vi "FGV_TE Controller.vi"(7 "Operation (Read)":T4, 8 "error in (no error)":errorcluster, 11 "FGV_TEC_IN":T1={"SVs"={"Unused"=0.0}, "PVs"={"FW & HW Versions"={"Device Type [I32]"=0, "Device Type [String]"="", "Firmware Version [I32]"=0, "Firmware Version [String]"="", "Hardware Version [I32]"=0, "Hardware Version [String]"="", "Serial No."=0}, "TEC Configuration"={"VISA resource name"="", "Device Address"=2}, "Object Target Temperature Source_CH1"=0, "Object Target Temperature Source_CH2"=0}, "Front Panel References"={"Main Loop Queue"=refnum, "meTEC_Device Type"=refnum, "meTEC_Serial No."=refnum, "meTEC_Hardware Version"=refnum, "meTEC_Firmware Version"=refnum, "meTEC_CH1_Object Target Temperature (ID 3000 / 50012) [°C]"=refnum, "meTEC_CH1_Live Set Current (ID 50001) [A]"=refnum, "meTEC_CH1_Live Set Voltage (ID 50002) [V]"=refnum, "meTEC_CH1_Live Enable (ID 50000)"=refnum, "meTEC_CH1_Input Selection (ID 2000)"=refnum, "meTEC_CH1_Object Target Temp. Source Sel. (ID 50011)"=refnum, "meTEC_CH2_Object Target Temperature (ID 3000 / 50012) [°C]"=refnum, "meTEC_CH2_Live Set Current (ID 50001) [A]"=refnum, "meTEC_CH2_Live Set Voltage (ID 50002) [V]"=refnum, "meTEC_CH2_Live Enable (ID 50000)"=refnum, "meTEC_CH2_Input Selection (ID 2000)"=refnum, "meTEC_CH2_Object Target Temp. Source Sel. (ID 50011)"=refnum, "meTEC_CH2_Object Temperature [°C]"=refnum, "meTEC_CH2_Sink Temperature [°C]"=refnum, "meTEC_CH2_Act. Output Current [A]"=refnum, "meTEC_CH2_Act. Output Voltage [V]"=refnum, "meTEC_CH2_Temperature Stability"=refnum, "Monitor Chart_CH2"=refnum, "meTEC_Initialize Device"=refnum}} caption="FGV_Rs Analyses_In") -> (0 "error out":errorcluster, 3 "FGV_TEC_OUT":T1={"SVs"={"Unused"=0.0}, "PVs"={"FW & HW Versions"={"Device Type [I32]"=0, "Device Type [String]"="", "Firmware Version [I32]"=0, "Firmware Version [String]"="", "Hardware Version [I32]"=0, "Hardware Version [String]"="", "Serial No."=0}, "TEC Configuration"={"VISA resource name"="", "Device Address"=2}, "Object Target Temperature Source_CH1"=0, "Object Target Temperature Source_CH2"=0}, "Front Panel References"={"Main Loop Queue"=refnum, "meTEC_Device Type"=refnum, "meTEC_Serial No."=refnum, "meTEC_Hardware Version"=refnum, "meTEC_Firmware Version"=refnum, "meTEC_CH1_Object Target Temperature (ID 3000 / 50012) [°C]"=refnum, "meTEC_CH1_Live Set Current (ID 50001) [A]"=refnum, "meTEC_CH1_Live Set Voltage (ID 50002) [V]"=refnum, "meTEC_CH1_Live Enable (ID 50000)"=refnum, "meTEC_CH1_Input Selection (ID 2000)"=refnum, "meTEC_CH1_Object Target Temp. Source Sel. (ID 50011)"=refnum, "meTEC_CH2_Object Target Temperature (ID 3000 / 50012) [°C]"=refnum, "meTEC_CH2_Live Set Current (ID 50001) [A]"=refnum, "meTEC_CH2_Live Set Voltage (ID 50002) [V]"=refnum, "meTEC_CH2_Live Enable (ID 50000)"=refnum, "meTEC_CH2_Input Selection (ID 2000)"=refnum, "meTEC_CH2_Object Target Temp. Source Sel. (ID 50011)"=refnum, "meTEC_CH2_Object Temperature [°C]"=refnum, "meTEC_CH2_Sink Temperature [°C]"=refnum, "meTEC_CH2_Act. Output Current [A]"=refnum, "meTEC_CH2_Act. Output Voltage [V]"=refnum, "meTEC_CH2_Temperature Stability"=refnum, "Monitor Chart_CH2"=refnum, "meTEC_Initialize Device"=refnum}} caption="FGV_Rs Analyses_Out")   [LabVIEW 2023]
uses:
  Type Defs/FGV_Operations.ctl
  Type Defs/FGV_TE Controller.ctl
  [meerstetter engineering TE Cooling]/TypeDefs/meTEC_Configuration.ctl
  Type Defs/FGV_Front Panel References.ctl
  Type Definitions/Main Loop Queue Data.ctl
  Type Definitions/Main Loop States.ctl
panel:
  # "Input"
  # "Output"
  # "PVs = Process Values"
  # "SVs = Set values / Values to be set"
  # "PVs = Process Values"
  # "SVs = Set values / Values to be set"
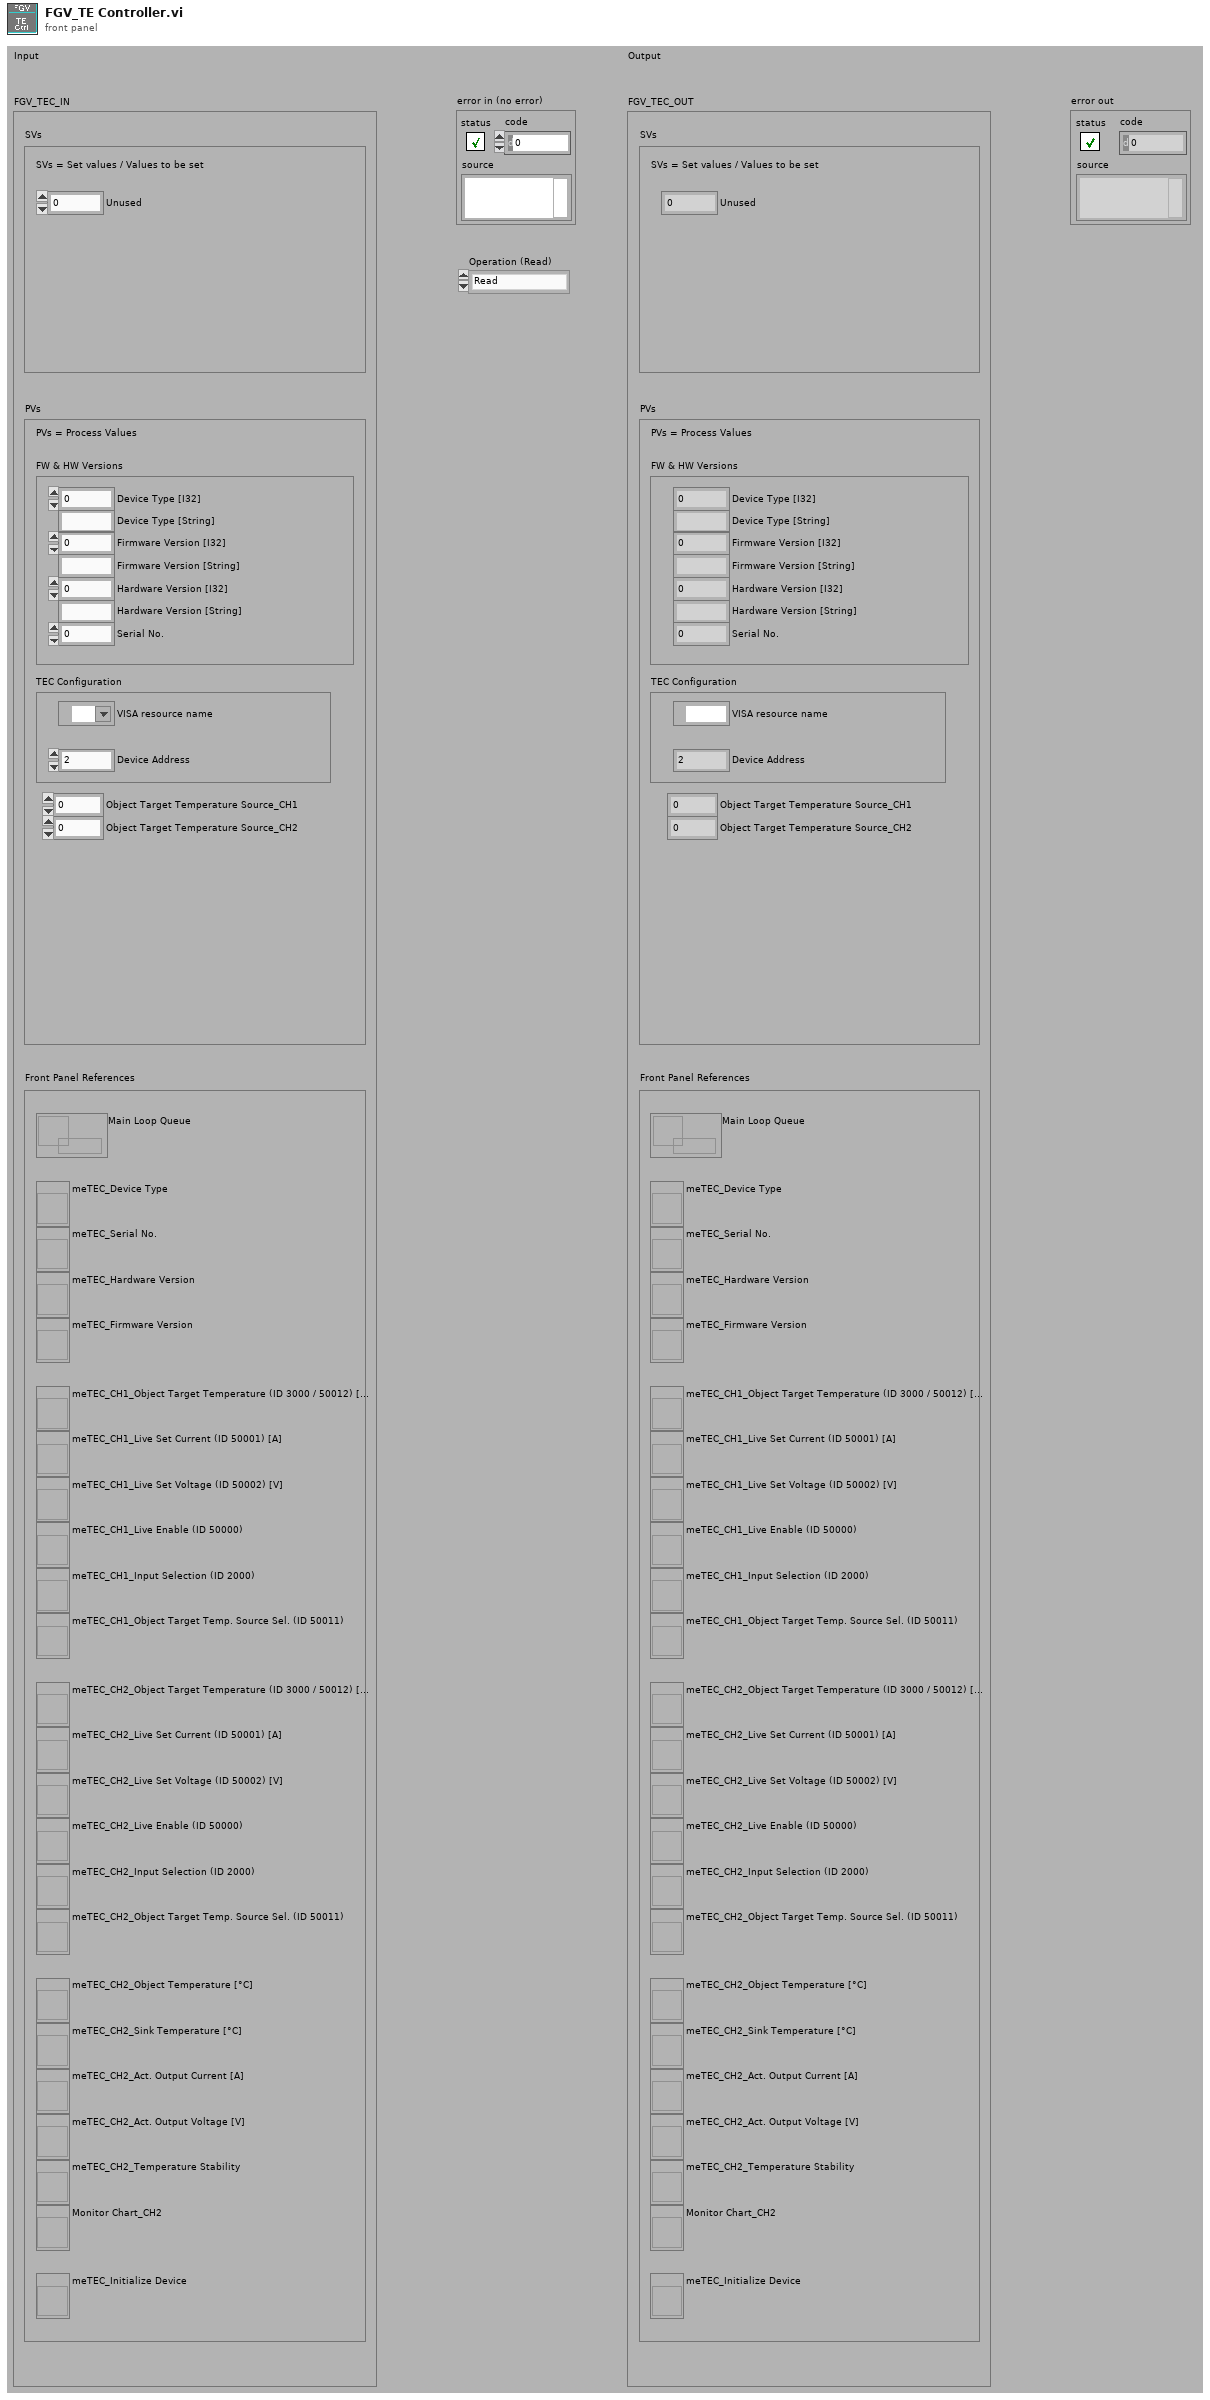
[diagram p1: front panel]
types:
  T1 = typedef "FGV_TE Controller.ctl" = cluster{"SVs":cluster{"Unused":dbl}, "PVs":cluster{"FW & HW Versions":cluster{"Device Type [I32]":i32, "Device Type [String]":string, "Firmware Version [I32]":i32, "Firmware Version [String]":string, "Hardware Version [I32]":i32, "Hardware Version [String]":string, "Serial No.":i32}, "TEC Configuration":T2, "Object Target Temperature Source_CH1":u8, "Object Target Temperature Source_CH2":u8}, "Front Panel References":T3}
  T2 = typedef "meTEC_Configuration.ctl" = cluster{"VISA resource name":refnum<visa-resource-name>, "Device Address":u16}
  T3 = typedef "FGV_Front Panel References.ctl" = cluster{"Main Loop Queue":refnum<queue>, "meTEC_Device Type":refnum<vi>, "meTEC_Serial No.":refnum<vi>, "meTEC_Hardware Version":refnum<vi>, "meTEC_Firmware Version":refnum<vi>, "meTEC_CH1_Object Target Temperature (ID 3000 / 50012) [°C]":refnum<vi>, "meTEC_CH1_Live Set Current (ID 50001) [A]":refnum<vi>, "meTEC_CH1_Live Set Voltage (ID 50002) [V]":refnum<vi>, "meTEC_CH1_Live Enable (ID 50000)":refnum<vi>, "meTEC_CH1_Input Selection (ID 2000)":refnum<vi>, "meTEC_CH1_Object Target Temp. Source Sel. (ID 50011)":refnum<vi>, "meTEC_CH2_Object Target Temperature (ID 3000 / 50012) [°C]":refnum<vi>, "meTEC_CH2_Live Set Current (ID 50001) [A]":refnum<vi>, "meTEC_CH2_Live Set Voltage (ID 50002) [V]":refnum<vi>, "meTEC_CH2_Live Enable (ID 50000)":refnum<vi>, "meTEC_CH2_Input Selection (ID 2000)":refnum<vi>, "meTEC_CH2_Object Target Temp. Source Sel. (ID 50011)":refnum<vi>, "meTEC_CH2_Object Temperature [°C]":refnum<vi>, "meTEC_CH2_Sink Temperature [°C]":refnum<vi>, "meTEC_CH2_Act. Output Current [A]":refnum<vi>, "meTEC_CH2_Act. Output Voltage [V]":refnum<vi>, "meTEC_CH2_Temperature Stability":refnum<vi>, "Monitor Chart_CH2":refnum<vi>, "meTEC_Initialize Device":refnum<vi>}
  T4 = typedef "FGV_Operations.ctl" = enum16{"Read", "Write"}
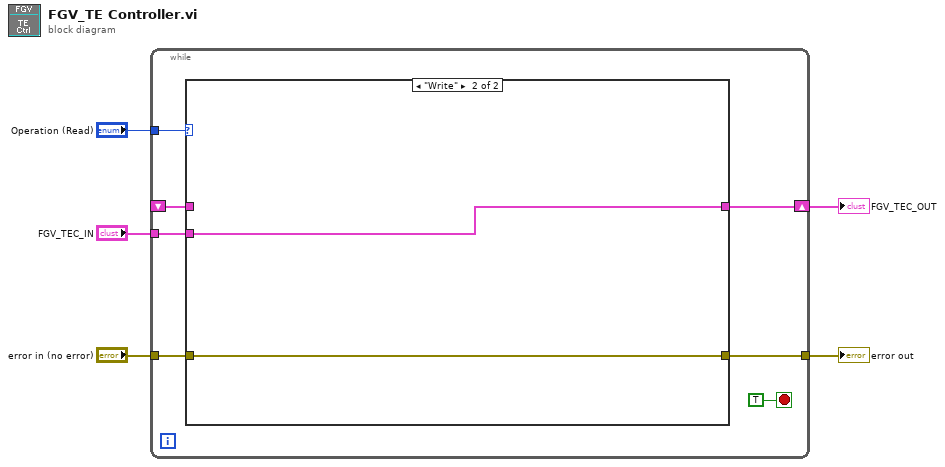
[diagram p0: block diagram]
diagram:
  n1 = while {
    shift-right: [w8] -> w2
    shift-left: _ -> [w10]
    tunnel: "error in (no error)" -> [w12]
    tunnel: [w11] -> w4
    tunnel: "FGV_TEC_IN" -> [w9]
    tunnel: "Operation (Read)" -> [w7]
    stop <- TRUE stop-if-true
    n2 = case shown="\"Write\"" w7 {
      tunnel: w10 -> [w14 _]
      tunnel: [w14 w15] -> w8
      tunnel: w12 -> [w13 w16]
      tunnel: [w13 w16] -> w11
      tunnel: w9 -> [_ w15]
      frame "Read", Default {
      }
      frame "Write" {
      }
    }
  }
  "error out" <- w4
  "FGV_TEC_OUT" <- w2
